vi "Read Tab Control.vi"(8 "error in (no error)":errorcluster, 11 "Function UI in":refnum<class "Controller UI.lvclass">) -> (0 "error out":errorcluster, 2 "Tab Control":refnum<vi>, 3 "Function UI out":refnum<class "Controller UI.lvclass">)   [LabVIEW 2016, in "Controller UI.lvlib" / "Controller UI.lvclass"]
uses:
  <userlib>/Common Components/Controller UI/Controller UI.lvclass
  <userlib>/Common Components/Controller UI/Controller UI.lvclass/Controller UI.ctl
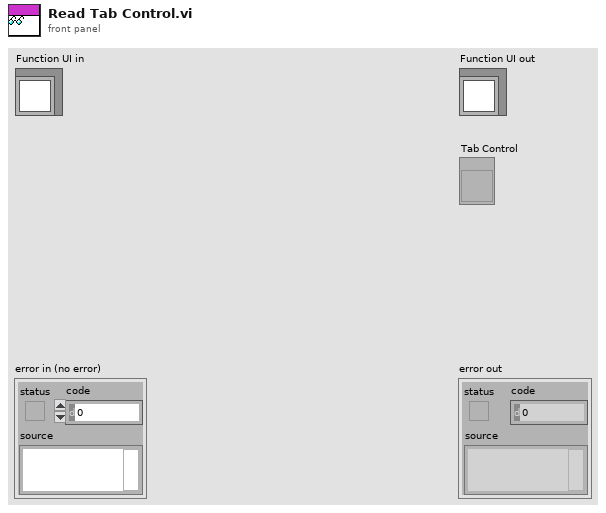
[diagram p1: front panel]
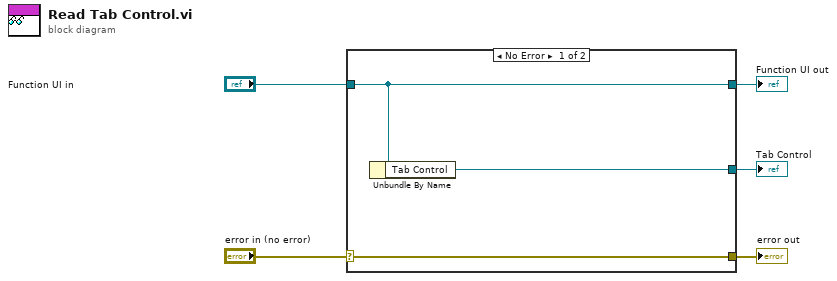
[diagram p0: block diagram]
diagram:
  n1 = case shown="No Error" "error in (no error)" {
    selector: "error in (no error)" -> [w8 w9]
    tunnel: [w8 w9] -> w4
    tunnel: [w7 w10] -> w2
    tunnel: "Function UI in" -> [w7 w10]
    tunnel: [w6 _] -> w1
    frame No Error {
      n2 = Unbundle By Name(w7) -> ("Tab Control"=w6:refnum<vi>)
    }
    frame Error {
    }
  }
  "error out" <- w4
  "Function UI out" <- w2
  "Tab Control" <- w1
